vi "N-664 Startup.vi"(0 "VISA Ref":refnum<visa-resource-name>, 11 "Error In":errorcluster) -> (4 "VISA Ref Dup":refnum<visa-resource-name>, 15 "Error Out":errorcluster)   [LabVIEW 2020]
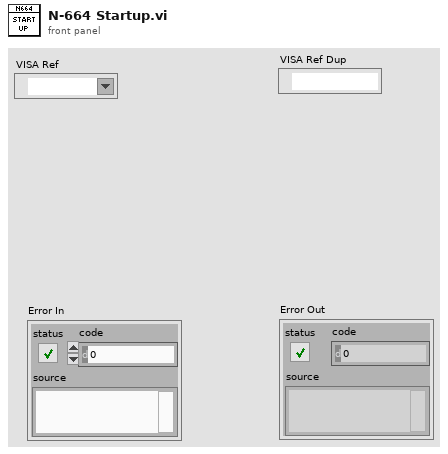
[diagram p1: front panel]
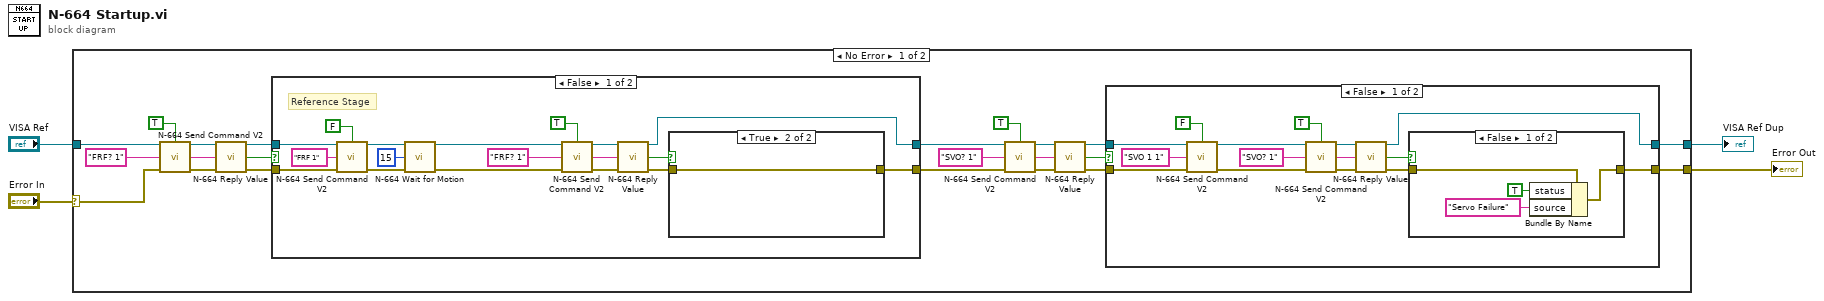
[diagram p0: block diagram]
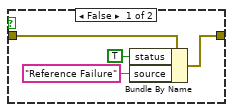
[diagram p4: hidden frame]
diagram:
  n1 = case shown="No Error" "Error In" {
    selector: "Error In" -> [w24 w74]
    tunnel: "VISA Ref" -> [w26 w75]
    tunnel: [w6 w75] -> w2
    tunnel: [w5 w74] -> w1
    frame No Error {
      n2 = call "N-664 Send Command V2.vi"("VISA Ref"=w26, "Wait for Reply (T)"=TRUE, "Command"="FRF? 1", "Error In"=w24) -> ("VISA Ref Dup"=w20:refnum<visa-resource-name>, "Reply"=w22:string, "Error Out"=w21:errorcluster)  [unwired: 8 in, 1 out]
      n3 = call "N-664 Reply Value.vi"("VISA Pass Thru"=w20, "Cmd Reply"=w22, "Error In"=w21) -> ("VISA Ref Dup"=w17:refnum<visa-resource-name>, "Bool"=w19:bool, "Error Out"=w18:errorcluster)  [unwired: 9 in, 1 out]
      n4 = case shown="False" w19 {
        tunnel: w18 -> [w65 w72]
        tunnel: w17 -> [w66 w73]
        tunnel: [w50 w73] -> w13
        tunnel: [w49 w72] -> w14
        frame False {
          # "Reference Stage"
          n5 = call "N-664 Send Command V2.vi"("VISA Ref"=w66, "Wait for Reply (T)"=FALSE, "Command"="FRF 1", "Error In"=w65) -> ("VISA Ref Dup"=w61:refnum<visa-resource-name>, "Error Out"=w62:errorcluster)  [unwired: 8 in, 2 out]
          n6 = call "N-664 Wait for Motion.vi"("VISA Ref"=w61, "Timeout (s)"=15, "Error In"=w62) -> ("VISA Ref Dup"=w54:refnum<visa-resource-name>, "Error Out"=w53:errorcluster)  [unwired: 11 in]
          n7 = call "N-664 Send Command V2.vi"("VISA Ref"=w54, "Wait for Reply (T)"=TRUE, "Command"="FRF? 1", "Error In"=w53) -> ("VISA Ref Dup"=w59:refnum<visa-resource-name>, "Reply"=w57:string, "Error Out"=w58:errorcluster)  [unwired: 8 in, 1 out]
          n8 = call "N-664 Reply Value.vi"("VISA Pass Thru"=w59, "Cmd Reply"=w57, "Error In"=w58) -> ("VISA Ref Dup"=w50:refnum<visa-resource-name>, "Bool"=w52:bool, "Error Out"=w51:errorcluster)  [unwired: 9 in, 1 out]
          n9 = case shown="True" w52 {
            tunnel: w51 -> [w70 w71]
            tunnel: [w67 w71] -> w49
            frame False {
              n10 = Bundle By Name(cluster=w70, "status"=TRUE, "source"="Reference Failure") -> (w67:errorcluster)
            }
            frame True {
            }
          }
        }
        frame True {
        }
      }
      n11 = call "N-664 Send Command V2.vi"("VISA Ref"=w13, "Wait for Reply (T)"=TRUE, "Command"="SVO? 1", "Error In"=w14) -> ("VISA Ref Dup"=w12:refnum<visa-resource-name>, "Reply"=w11:string, "Error Out"=w10:errorcluster)  [unwired: 8 in, 1 out]
      n12 = call "N-664 Reply Value.vi"("VISA Pass Thru"=w12, "Cmd Reply"=w11, "Error In"=w10) -> ("VISA Ref Dup"=w8:refnum<visa-resource-name>, "Bool"=w9:bool, "Error Out"=w7:errorcluster)  [unwired: 9 in, 1 out]
      n13 = case shown="False" w9 {
        tunnel: w8 -> [w39 w48]
        tunnel: w7 -> [w38 w47]
        tunnel: [w28 w47] -> w5
        tunnel: [w27 w48] -> w6
        frame False {
          n14 = call "N-664 Send Command V2.vi"("VISA Ref"=w39, "Wait for Reply (T)"=FALSE, "Command"="SVO 1 1", "Error In"=w38) -> ("VISA Ref Dup"=w32:refnum<visa-resource-name>, "Error Out"=w31:errorcluster)  [unwired: 8 in, 2 out]
          n15 = call "N-664 Send Command V2.vi"("VISA Ref"=w32, "Wait for Reply (T)"=TRUE, "Command"="SVO? 1", "Error In"=w31) -> ("VISA Ref Dup"=w35:refnum<visa-resource-name>, "Reply"=w36:string, "Error Out"=w37:errorcluster)  [unwired: 8 in, 1 out]
          n16 = call "N-664 Reply Value.vi"("VISA Pass Thru"=w35, "Cmd Reply"=w36, "Error In"=w37) -> ("VISA Ref Dup"=w27:refnum<visa-resource-name>, "Bool"=w30:bool, "Error Out"=w29:errorcluster)  [unwired: 9 in, 1 out]
          n17 = case shown="False" w30 {
            tunnel: w29 -> [w45 w46]
            tunnel: [w42 w46] -> w28
            frame False {
              n18 = Bundle By Name(cluster=w45, "status"=TRUE, "source"="Servo Failure") -> (w42:errorcluster)
            }
            frame True {
            }
          }
        }
        frame True {
        }
      }
    }
    frame Error {
    }
  }
  "Error Out" <- w1
  "VISA Ref Dup" <- w2
